vi "Query Self-Alignment Last Valid Date Time.vi"(8 "error in (no error)":errorcluster, 11 "VISA resource name":refnum<visa-resource-name>) -> (0 "error out":errorcluster, 1 "Time IQ":string, 2 "Date IQ":string, 3 "VISA resource name out":refnum<visa-resource-name>, 4 "Date Level":string, 5 "Time Level":string)   [LabVIEW 2015, in "Rohde&Schwarz CMXP Base.lvlib"]
doc: "Queries the date and time of the last successful execution of the self-alignment procedure. The information is returned for the measurement modes \"IQ\" and \"Level\": <Date>IQ, <Time>IQ, <Date>level, <Time>level\n\nAttribute:\nRSCMXPBASE_ATTR_QUERY_LAST_SUCCESFULL_PROCEDURE\n\nRemote-control command:\nFETCh:BASE:SALignment:LVALid?"
uses:
  <instrlib>/Rohde&Schwarz CMXP Base/Rohde&Schwarz CMXP Base.lvlib
  <instrlib>/Rohde&Schwarz CMXP Base/Private/rsidr_core.llb/rsidr_core.lvlib
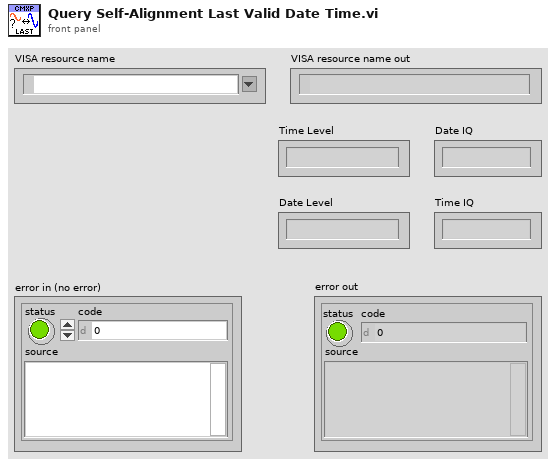
[diagram p1: front panel]
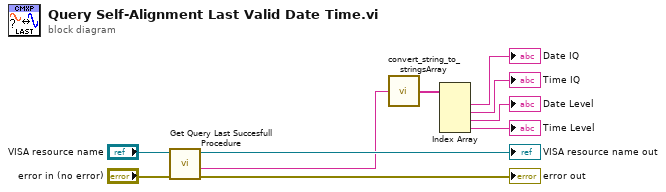
[diagram p0: block diagram]
diagram:
  n1 = call "Get Query Last Succesfull Procedure"("error in (no error)"="error in (no error)", "instrument handle"="VISA resource name") -> ("error out"=→"error out":errorcluster, "Query Last Succesfull Procedure"=w4:string, "instrument handle out"=→"VISA resource name out":refnum<visa-resource-name>)  [unwired: 7 in]
  n2 = call <instrlib>:"convert_string_to_stringsArray.vi"("String in"=w4) -> ("string array out"=w6:string[])  [unwired: 3 in, 1 out]
  n3 = Index Array(array=w6) -> (element #1=→"Date IQ":string, element #2=→"Time IQ":string, element #3=→"Date Level":string, element #4=→"Time Level":string)  [unwired: 4 in]
